vi "核查数据发送(子VI).vi"(8 "错误输入":errorcluster) -> (0 "错误输出":errorcluster)   [LabVIEW 2016, in "数据传输系统.lvlib"]
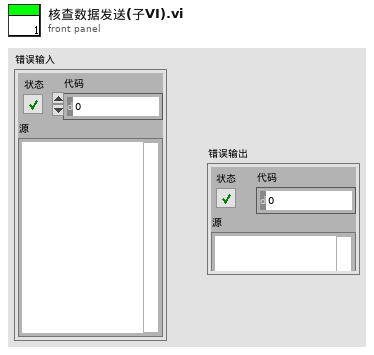
[diagram p1: front panel]
types:
  T1 = enum16{"质控数据", "操作日志", "仪器参数", "系统状态", "运行模式", "测量周期", "超标留样", "报警信息", "环境参数"}
  T2 = enum16{"空白测试", "跨度核查", "标样核查", "加标回收", "平行样", "集成干预"}
  T3 = cluster{"氨氮零点核查索引起始时间":string, "总磷零点核查索引起始时间":string, "总氮零点核查索引起始时间":string, "CODMn零点核查索引起始时间":string, "CODCr零点核查索引起始时间":string, "亚硝酸盐零点核查索引起始时间":string, "硫化物零点核查索引起始时间":string, "ORP零点核查索引起始时间":string}
  T4 = cluster{"[0]":string, "[1]":string, "[2]":string, "[3]":string, "[4]":string, "[5]":string, "[6]":string, "[7]":string}
  T5 = cluster{"PH":string[][], "CODCr":string[][], "氨氮":string[][], "CODMn":string[][], "总氮":string[][], "总磷":string[][], "电导率":string[][], "水温":string[][], "DO":string[][], "浊度":string[][], "叶绿素":string[][], "藻密度":string[][], "铜":string[][], "盐度":string[][], "水位":string[][], "流速":string[][], "瞬时流量":string[][], "累积流量":string[][], "亚硝酸盐":string[][], "硫化物":string[][], "ORP":string[][], "铅":string[][], "镉":string[][], "锌":string[][], "镍":string[][], "锰":string[][], "汞":string[][], "气温":string[][], "气压":string[][], "风速":string[][], "风向":string[][]}
  T6 = cluster{"氨氮跨度核查索引起始时间":string, "总磷跨度核查索引起始时间":string, "总氮跨度核查索引起始时间":string, "CODMn跨度核查索引起始时间":string, "CODCr跨度核查索引起始时间":string, "亚硝酸盐跨度核查索引起始时间":string, "硫化物跨度核查索引起始时间":string, "ORP跨度核查索引起始时间":string}
  T7 = cluster{"氨氮标样核查索引起始时间":string, "总磷标样核查索引起始时间":string, "总氮标样核查索引起始时间":string, "CODMn标样核查索引起始时间":string, "CODCr标样核查索引起始时间":string, "DO标样核查索引起始时间":string, "PH标样核查索引起始时间":string, "比电导率标样核查索引起始时间":string, "水温标样核查索引起始时间":string, "浊度标样核查索引起始时间":string, "叶绿素a标样核查索引起始时间":string, "藻密度标样核查索引起始时间":string, "亚硝酸盐标样核查索引起始时间":string, "硫化物标样核查索引起始时间":string, "ORP标样核查索引起始时间":string}
  T8 = cluster{"[0]":string, "[1]":string, "[2]":string, "[3]":string, "[4]":string, "[5]":string, "[6]":string, "[7]":string, "[8]":string, "[9]":string, "[10]":string, "[11]":string, "[12]":string, "[13]":string, "[14]":string}
  T9 = cluster{"氨氮加标回收索引起始时间":string, "总磷加标回收索引起始时间":string, "总氮加标回收索引起始时间":string, "CODMn加标回收索引起始时间":string, "CODCr加标回收索引起始时间":string}
  T10 = cluster{"[0]":string, "[1]":string, "[2]":string, "[3]":string, "[4]":string}
  T11 = cluster{"氨氮平行样索引起始时间":string, "总磷平行样索引起始时间":string, "总氮平行样索引起始时间":string, "CODMn平行样索引起始时间":string, "CODCr平行样索引起始时间":string}
  T12 = cluster{"氨氮集成干预索引起始时间":string, "总磷集成干预索引起始时间":string, "总氮集成干预索引起始时间":string, "CODMn集成干预索引起始时间":string, "CODCr集成干预索引起始时间":string, "DO集成干预索引起始时间":string, "PH集成干预索引起始时间":string, "比电导率集成干预索引起始时间":string, "水温集成干预索引起始时间":string, "浊度集成干预索引起始时间":string, "叶绿素a集成干预索引起始时间":string, "藻密度集成干预索引起始时间":string, "亚硝酸盐集成干预索引起始时间":string, "硫化物集成干预索引起始时间":string, "ORP集成干预索引起始时间":string}
  T13 = cluster{"氨氮仪器日志索引起始时间":string, "总磷仪器日志索引起始时间":string, "总氮仪器日志索引起始时间":string, "CODMn仪器日志索引起始时间":string, "CODCr仪器日志索引起始时间":string, "系统仪器日志索引起始时间":string}
  T14 = cluster{"[0]":string, "[1]":string, "[2]":string, "[3]":string, "[4]":string, "[5]":string}
  T15 = cluster{"氨氮仪器参数索引起始时间":string, "总磷仪器参数索引起始时间":string, "总氮仪器参数索引起始时间":string, "CODMn仪器参数索引起始时间":string, "CODCr仪器参数索引起始时间":string, "DO仪器参数索引起始时间":string, "PH仪器参数索引起始时间":string, "比电导率仪器参数索引起始时间":string, "水温仪器参数索引起始时间":string, "浊度仪器参数索引起始时间":string, "叶绿素a仪器参数索引起始时间":string, "藻密度仪器参数索引起始时间":string, "ORP仪器参数索引起始时间":string}
  T16 = cluster{"[0]":string, "[1]":string, "[2]":string, "[3]":string, "[4]":string, "[5]":string, "[6]":string, "[7]":string, "[8]":string, "[9]":string, "[10]":string, "[11]":string, "[12]":string}
  T17 = cluster{"氨氮报警信息索引起始时间":string, "总磷报警信息索引起始时间":string, "总氮报警信息索引起始时间":string, "CODMn报警信息索引起始时间":string, "CODCr报警信息索引起始时间":string, "DO报警信息索引起始时间":string, "PH报警信息索引起始时间":string, "比电导率报警信息索引起始时间":string, "水温报警信息索引起始时间":string, "浊度报警信息索引起始时间":string, "叶绿素报警信息索引起始时间":string, "系统报警信息索引起始时间":string}
  T18 = cluster{"[0]":string, "[1]":string, "[2]":string, "[3]":string, "[4]":string, "[5]":string, "[6]":string, "[7]":string, "[8]":string, "[9]":string, "[10]":string, "[11]":string}
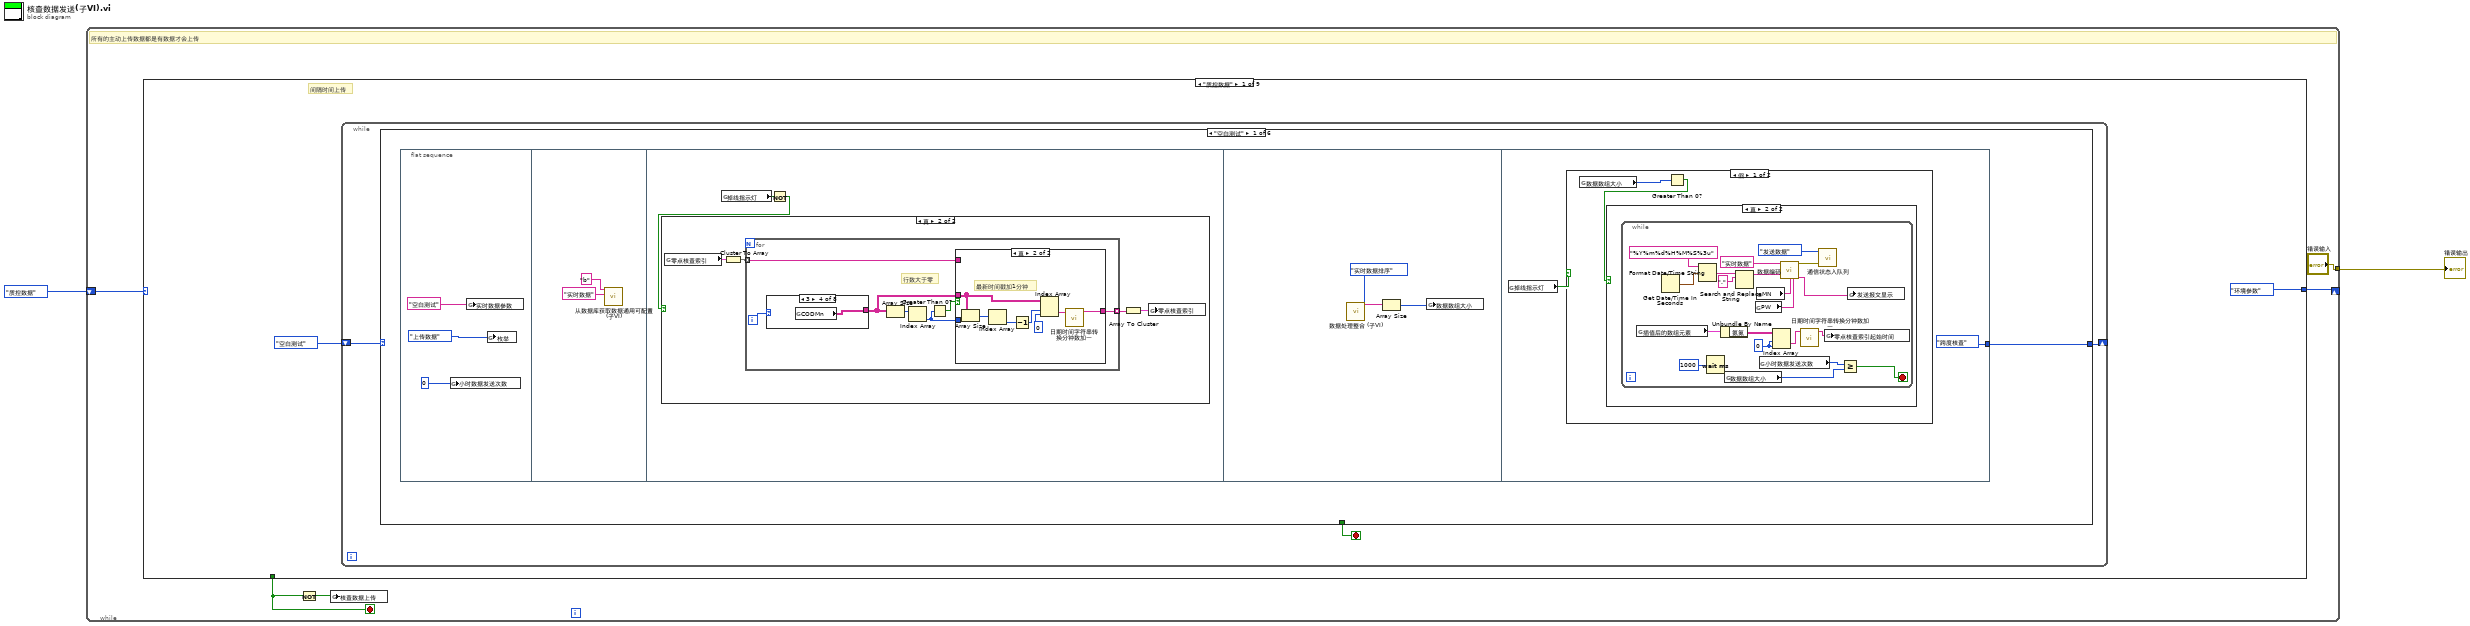
[diagram p0: block diagram]
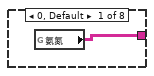
[diagram p3: hidden frame]
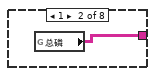
[diagram p4: hidden frame]
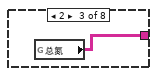
[diagram p5: hidden frame]
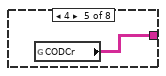
[diagram p6: hidden frame]
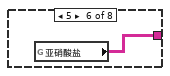
[diagram p7: hidden frame]
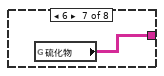
[diagram p8: hidden frame]
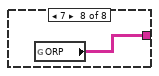
[diagram p9: hidden frame]
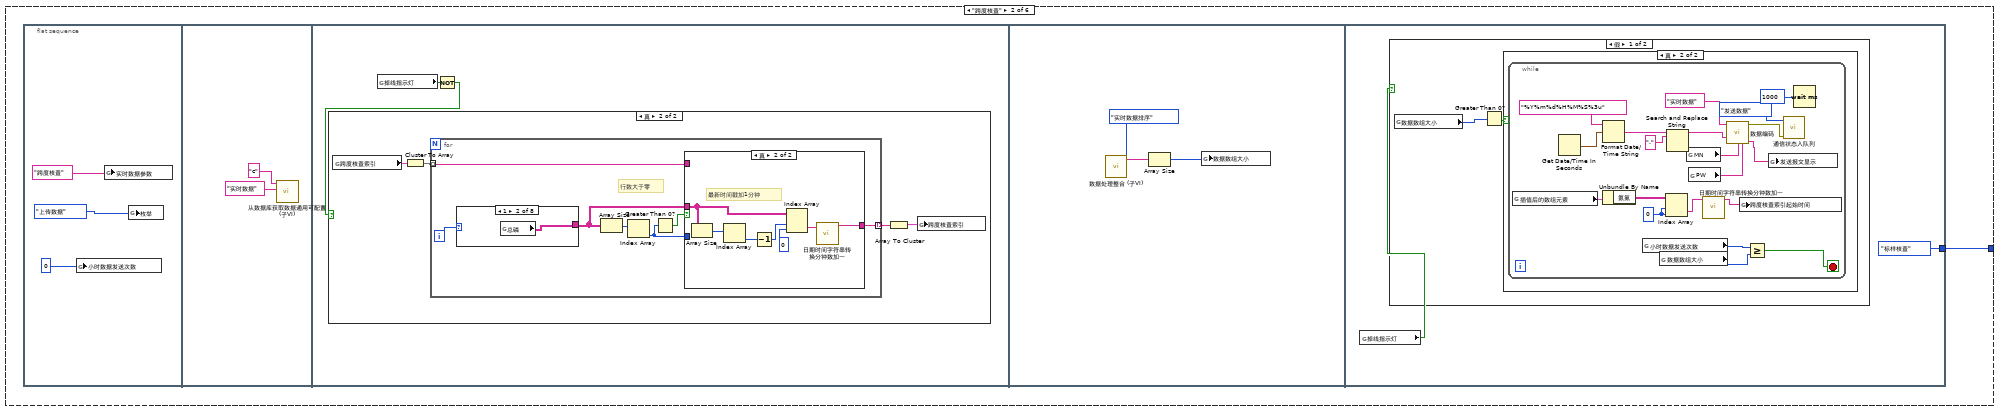
[diagram p13: hidden frame]
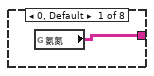
[diagram p15: hidden frame]
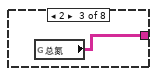
[diagram p16: hidden frame]
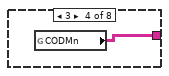
[diagram p17: hidden frame]
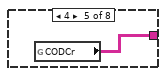
[diagram p18: hidden frame]
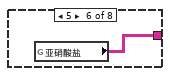
[diagram p19: hidden frame]
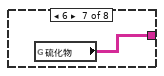
[diagram p20: hidden frame]
diagram:
  n1 = while "While循环" {
    shift-right: [w6] -> _
    shift-left: T1."质控数据" -> [w7]
    tunnel: ["错误输入"] -> w1
    stop <- w4 stop-if-true
    # "所有的主动上传数据都是有数据才会上传"
    n2 = case shown="\"质控数据\"" w7 {
      tunnel: [T1."环境参数" T1."仪器参数" T1."系统状态" T1."运行模式" T1."测量周期" T1."超标留样" T1."报警信息" T1."环境参数" T1."环境参数"] -> w6
      tunnel: [_ _ _ _ _ _ _ _ TRUE] -> w4
      frame "质控数据" {
        # "间隔时间上传"
        n3 = while {
          shift-right: [w10] -> _
          shift-left: T2."空白测试" -> [w11]
          stop <- w12 stop-if-true
          n4 = case shown="\"空白测试\"" w11 {
            tunnel: [_ _ _ _ _ TRUE] -> w12
            tunnel: [w13 w75 w137 w206 w267 w321] -> w10
            frame "空白测试" {
              n5 = flat-sequence {
                tunnel: [T2."跨度核查"] -> w13
                frame #0 {
                  n6 = global write "全局 小时数据发送次数.vi" "小时数据发送次数"(0 ("小时数据发送次数")) -> ()
                  n7 = global write "全局 实时数据参数.vi" "实时数据参数"("空白测试") -> ()
                  n8 = global write "全局1.vi" "枚举"(enum16{"返回请求应答", "上传数据", "返回执行结果"}."上传数据" ("枚举")) -> ()
                }
                frame #1 {
                  n9 = call "从数据库获取数据通用可配置(子VI).vi"("table输入"="实时数据" ("新元素/子数组"), "列队名（唯一）"="b") -> ()  [unwired: 8 in, 2 out]
                }
                frame #2 {
                  n10 = global read "全局 数据发送重叠.vi" "掉线指示灯"() -> (w20:bool)
                  n11 = Not(x=w20) -> (.not. x?=w19:bool)
                  n12 = case shown="真" w19 {
                    frame False {
                    }
                    frame True {
                      n13 = global read "全局 时间2.vi" "零点核查索引"() -> (w24:T3)
                      n14 = Cluster To Array(cluster=w24) -> (array=w23:string[])
                      n15 = for {
                        tunnel: [w26] -> w22 mode=indexing
                        tunnel: w23 -> [w25] mode=indexing
                        i -> [w27]
                        # "行数大于零"
                        n16 = case shown="3" w27 {
                          tunnel: [w32 w33 w34 w35 w36 w37 w38 w39] -> w28
                          frame 0, Default {
                            n17 = global read "全局 所有参数.vi" "氨氮"() -> (w32:string[][])
                          }
                          frame 1 {
                            n18 = global read "全局 所有参数.vi" "总磷"() -> (w33:string[][])
                          }
                          frame 2 {
                            n19 = global read "全局 所有参数.vi" "总氮"() -> (w34:string[][])
                          }
                          frame 3 {
                            n20 = global read "全局 所有参数.vi" "CODMn"() -> (w35:string[][])
                          }
                          frame 4 {
                            n21 = global read "全局 所有参数.vi" "CODCr"() -> (w36:string[][])
                          }
                          frame 5 {
                            n22 = global read "全局 所有参数.vi" "亚硝酸盐"() -> (w37:string[][])
                          }
                          frame 6 {
                            n23 = global read "全局 所有参数.vi" "硫化物"() -> (w38:string[][])
                          }
                          frame 7 {
                            n24 = global read "全局 所有参数.vi" "ORP"() -> (w39:string[][])
                          }
                        }
                        n25 = Array Size(array=w28) -> (size(s)=w30:i32[])
                        n26 = Index Array(array=w30) -> (element=w29:i32)  [unwired: 1 in]
                        n27 = Greater Than 0?(x=w29) -> (x > 0?=w31:bool)
                        n28 = case shown="真" w31 {
                          tunnel: w29 -> [_ _]
                          tunnel: w28 -> [_ w43]
                          tunnel: [w40 w41] -> w26
                          tunnel: w25 -> [w40 _]
                          frame False {
                          }
                          frame True {
                            # "最新时间戳加1分钟"
                            n29 = Array Size(array=w43) -> (size(s)=w46:i32[])
                            n30 = Index Array(array=w46) -> (element=w45:i32)  [unwired: 1 in]
                            n31 = Decrement(x=w45) -> (x-1=w44:i32)
                            n32 = Index Array(array=w43, index (row)=w44, index (col)=0 ("禁用的索引 (列)")) -> (element=w47:string)
                            n33 = call "日期时间字符串转换分钟数加一.vi"("data[0]"=w47) -> ("日期/时间字符串"=w41:string)  [unwired: 10 in]
                          }
                        }
                      }
                      n34 = Array To Cluster(array=w22) -> (cluster=w21:T4)
                      n35 = global write "全局 时间2.vi" "零点核查索引"(w21) -> ()
                    }
                  }
                }
                frame #3 {
                  n36 = call "数据处理整合 (子VI).vi"("枚举"=enum16{"实时数据排序", "小时数据排序"}."实时数据排序") -> ("已排序的数组"=w50:string[])  [unwired: 10 in]
                  n37 = Array Size(array=w50) -> (size(s)=w49:i32)
                  n38 = global write "全局 数据数组大小.vi" "数据数组大小"(w49) -> ()
                }
                frame #4 {
                  n39 = global read "全局 数据发送重叠.vi" "掉线指示灯"() -> (w52:bool)
                  n40 = case shown="假" w52 {
                    frame False {
                      n41 = global read "全局 数据数组大小.vi" "数据数组大小"() -> (w54:i32)
                      n42 = Greater Than 0?(x=w54) -> (x > 0?=w53:bool)
                      n43 = case shown="真" w53 {
                        frame False {
                        }
                        frame True {
                          n44 = while {
                            stop <- w60 stop-if-true
                            w69 = 0 ("禁用的索引 (列)")
                            n45 = global read "插值后的新数组.vi" "插值后的数组元素"() -> (w73:T5)
                            n46 = Get Date/Time In Seconds() -> (seconds since 1Jan1904=w58:timestamp)
                            n47 = Format Date/Time String(time format string (%c)="%Y%m%d%H%M%S%3u" ("时间格式字符串(%c)"), seconds (now)=w58) -> (date/time string=w57:string)  [unwired: 1 in]
                            n48 = Wait (ms)(milliseconds to wait=u32 1000 ("等待时间（毫秒）")) -> ()  [unwired: 1 out]
                            n49 = Unbundle By Name(w73) -> ("氨氮"=w72:string[][])
                            n50 = global read "全局 数据数组大小.vi" "数据数组大小"() -> (w63:i32)
                            n51 = Search and Replace String(input string=w57, search string="." ("搜索字符串")) -> (result string=w55:string)  [unwired: 6 in, 3 out]
                            n52 = global read "断电保存全局.vi" "PW"() -> (w65:string)
                            n53 = global read "断电保存全局.vi" "MN"() -> (w66:string)
                            n54 = global read "全局 小时数据发送次数.vi" "小时数据发送次数"() -> (w61:i32)
                            n55 = Index Array(array=w72, index (row)=w69, index (col)=w69) -> (element=w71:string)
                            n56 = call "数据编码.vi"("table输入"="实时数据" ("新元素/子数组"), "QN"=w55, "MN"=w66, "PW"=w65) -> ("错误常量"=w64:errorcluster, "通讯包字符串"=w68:string)  [unwired: 10 in]
                            n57 = call "日期时间字符串转换分钟数加一.vi"("data[0]"=w71) -> ("日期/时间字符串"=w70:string)  [unwired: 10 in]
                            n58 = call "通信状态入队列.vi"("错误输入（无错误）"=w64, "枚举"=enum16{"打开连接", "发送数据", "读取数据", "数据处理", "关闭连接"}."发送数据") -> ()  [unwired: 9 in, 1 out]
                            n59 = global write "全局 时间2.vi" "零点核查索引起始时间"(w70) -> ()
                            n60 = Greater Or Equal?(x=w61, y=w63) -> (x >= y?=w60:bool)
                            n61 = global write "全局1.vi" "发送报文显示"(w68) -> ()
                          }
                        }
                      }
                    }
                    frame True {
                    }
                  }
                }
              }
            }
            frame "跨度核查" {
              n62 = flat-sequence {
                tunnel: [T2."标样核查"] -> w75
                frame #0 {
                  n63 = global write "全局 小时数据发送次数.vi" "小时数据发送次数"(0 ("小时数据发送次数")) -> ()
                  n64 = global write "全局 实时数据参数.vi" "实时数据参数"("跨度核查") -> ()
                  n65 = global write "全局1.vi" "枚举"(enum16{"返回请求应答", "上传数据", "返回执行结果"}."上传数据" ("枚举")) -> ()
                }
                frame #1 {
                  n66 = call "从数据库获取数据通用可配置(子VI).vi"("table输入"="实时数据" ("新元素/子数组"), "列队名（唯一）"="c") -> ()  [unwired: 8 in, 2 out]
                }
                frame #2 {
                  n67 = global read "全局 数据发送重叠.vi" "掉线指示灯"() -> (w82:bool)
                  n68 = Not(x=w82) -> (.not. x?=w81:bool)
                  n69 = case shown="真" w81 {
                    frame False {
                    }
                    frame True {
                      n70 = global read "全局 时间2.vi" "跨度核查索引"() -> (w86:T6)
                      n71 = Cluster To Array(cluster=w86) -> (array=w85:string[])
                      n72 = for {
                        tunnel: [w88] -> w84 mode=indexing
                        tunnel: w85 -> [w87] mode=indexing
                        i -> [w89]
                        # "行数大于零"
                        n73 = case shown="1" w89 {
                          tunnel: [w94 w95 w96 w97 w98 w99 w100 w101] -> w90
                          frame 0, Default {
                            n74 = global read "全局 所有参数.vi" "氨氮"() -> (w94:string[][])
                          }
                          frame 1 {
                            n75 = global read "全局 所有参数.vi" "总磷"() -> (w95:string[][])
                          }
                          frame 2 {
                            n76 = global read "全局 所有参数.vi" "总氮"() -> (w96:string[][])
                          }
                          frame 3 {
                            n77 = global read "全局 所有参数.vi" "CODMn"() -> (w97:string[][])
                          }
                          frame 4 {
                            n78 = global read "全局 所有参数.vi" "CODCr"() -> (w98:string[][])
                          }
                          frame 5 {
                            n79 = global read "全局 所有参数.vi" "亚硝酸盐"() -> (w99:string[][])
                          }
                          frame 6 {
                            n80 = global read "全局 所有参数.vi" "硫化物"() -> (w100:string[][])
                          }
                          frame 7 {
                            n81 = global read "全局 所有参数.vi" "ORP"() -> (w101:string[][])
                          }
                        }
                        n82 = Array Size(array=w90) -> (size(s)=w92:i32[])
                        n83 = Index Array(array=w92) -> (element=w91:i32)  [unwired: 1 in]
                        n84 = Greater Than 0?(x=w91) -> (x > 0?=w93:bool)
                        n85 = case shown="真" w93 {
                          tunnel: w91 -> [_ _]
                          tunnel: w90 -> [_ w105]
                          tunnel: [w102 w103] -> w88
                          tunnel: w87 -> [w102 _]
                          frame False {
                          }
                          frame True {
                            # "最新时间戳加1分钟"
                            n86 = Array Size(array=w105) -> (size(s)=w108:i32[])
                            n87 = Index Array(array=w108) -> (element=w107:i32)  [unwired: 1 in]
                            n88 = Decrement(x=w107) -> (x-1=w106:i32)
                            n89 = Index Array(array=w105, index (row)=w106, index (col)=0 ("禁用的索引 (列)")) -> (element=w109:string)
                            n90 = call "日期时间字符串转换分钟数加一.vi"("data[0]"=w109) -> ("日期/时间字符串"=w103:string)  [unwired: 10 in]
                          }
                        }
                      }
                      n91 = Array To Cluster(array=w84) -> (cluster=w83:T4)
                      n92 = global write "全局 时间2.vi" "跨度核查索引"(w83) -> ()
                    }
                  }
                }
                frame #3 {
                  n93 = call "数据处理整合 (子VI).vi"("枚举"=enum16{"实时数据排序", "小时数据排序"}."实时数据排序") -> ("已排序的数组"=w112:string[])  [unwired: 10 in]
                  n94 = Array Size(array=w112) -> (size(s)=w111:i32)
                  n95 = global write "全局 数据数组大小.vi" "数据数组大小"(w111) -> ()
                }
                frame #4 {
                  n96 = global read "全局 数据发送重叠.vi" "掉线指示灯"() -> (w114:bool)
                  n97 = case shown="假" w114 {
                    frame False {
                      n98 = global read "全局 数据数组大小.vi" "数据数组大小"() -> (w116:i32)
                      n99 = Greater Than 0?(x=w116) -> (x > 0?=w115:bool)
                      n100 = case shown="真" w115 {
                        frame False {
                        }
                        frame True {
                          n101 = while {
                            stop <- w122 stop-if-true
                            w131 = 0 ("禁用的索引 (列)")
                            n102 = global read "插值后的新数组.vi" "插值后的数组元素"() -> (w135:T5)
                            n103 = Get Date/Time In Seconds() -> (seconds since 1Jan1904=w120:timestamp)
                            n104 = Format Date/Time String(time format string (%c)="%Y%m%d%H%M%S%3u" ("时间格式字符串(%c)"), seconds (now)=w120) -> (date/time string=w119:string)  [unwired: 1 in]
                            n105 = Unbundle By Name(w135) -> ("氨氮"=w134:string[][])
                            n106 = global read "全局 小时数据发送次数.vi" "小时数据发送次数"() -> (w123:i32)
                            n107 = global read "全局 数据数组大小.vi" "数据数组大小"() -> (w124:i32)
                            n108 = Index Array(array=w134, index (row)=w131, index (col)=w131) -> (element=w133:string)
                            n109 = Search and Replace String(input string=w119, search string="." ("搜索字符串")) -> (result string=w117:string)  [unwired: 6 in, 3 out]
                            n110 = global read "断电保存全局.vi" "MN"() -> (w129:string)
                            n111 = global read "断电保存全局.vi" "PW"() -> (w128:string)
                            n112 = call "日期时间字符串转换分钟数加一.vi"("data[0]"=w133) -> ("日期/时间字符串"=w132:string)  [unwired: 10 in]
                            n113 = call "数据编码.vi"("table输入"="实时数据" ("新元素/子数组"), "QN"=w117, "MN"=w129, "PW"=w128) -> ("错误常量"=w126:errorcluster, "通讯包字符串"=w127:string)  [unwired: 10 in]
                            n114 = global write "全局 时间2.vi" "跨度核查索引起始时间"(w132) -> ()
                            n115 = Greater Or Equal?(x=w123, y=w124) -> (x >= y?=w122:bool)
                            n116 = global write "全局1.vi" "发送报文显示"(w127) -> ()
                            n117 = call "通信状态入队列.vi"("错误输入（无错误）"=w126, "枚举"=enum16{"打开连接", "发送数据", "读取数据", "数据处理", "关闭连接"}."发送数据") -> ()  [unwired: 9 in, 1 out]
                            n118 = Wait (ms)(milliseconds to wait=u32 1000 ("等待时间（毫秒）")) -> ()  [unwired: 1 out]
                          }
                        }
                      }
                    }
                    frame True {
                    }
                  }
                }
              }
            }
            frame "标样核查" {
              n119 = flat-sequence {
                tunnel: [T2."加标回收"] -> w137
                frame #0 {
                  n120 = global write "全局 小时数据发送次数.vi" "小时数据发送次数"(0 ("小时数据发送次数")) -> ()
                  n121 = global write "全局 实时数据参数.vi" "实时数据参数"("核查数据") -> ()
                  n122 = global write "全局1.vi" "枚举"(enum16{"返回请求应答", "上传数据", "返回执行结果"}."上传数据" ("枚举")) -> ()
                }
                frame #1 {
                  n123 = call "从数据库获取数据通用可配置(子VI).vi"("table输入"="实时数据" ("新元素/子数组"), "列队名（唯一）"="n") -> ()  [unwired: 8 in, 2 out]
                }
                frame #2 {
                  n124 = global read "全局 数据发送重叠.vi" "掉线指示灯"() -> (w144:bool)
                  n125 = Not(x=w144) -> (.not. x?=w143:bool)
                  n126 = case shown="真" w143 {
                    frame False {
                    }
                    frame True {
                      n127 = global read "全局 时间2.vi" "标样核查索引"() -> (w148:T7)
                      n128 = Cluster To Array(cluster=w148) -> (array=w147:string[])
                      n129 = for {
                        tunnel: [w150] -> w145 mode=indexing
                        tunnel: w147 -> [w149] mode=indexing
                        i -> [w151]
                        # "行数大于零"
                        n130 = case shown="0, 默认" w151 {
                          tunnel: [w156 w157 w158 w159 w160 w161 w162 w163 w164 w165 w166 w167 w168 w169 w170] -> w152
                          frame 0, Default {
                            n131 = global read "全局 所有参数.vi" "氨氮"() -> (w156:string[][])
                          }
                          frame 1 {
                            n132 = global read "全局 所有参数.vi" "总磷"() -> (w157:string[][])
                          }
                          frame 2 {
                            n133 = global read "全局 所有参数.vi" "总氮"() -> (w158:string[][])
                          }
                          frame 3 {
                            n134 = global read "全局 所有参数.vi" "CODMn"() -> (w159:string[][])
                          }
                          frame 4 {
                            n135 = global read "全局 所有参数.vi" "CODCr"() -> (w160:string[][])
                          }
                          frame 5 {
                            n136 = global read "全局 所有参数.vi" "DO"() -> (w161:string[][])
                          }
                          frame 6 {
                            n137 = global read "全局 所有参数.vi" "PH"() -> (w162:string[][])
                          }
                          frame 7 {
                            n138 = global read "全局 所有参数.vi" "电导率"() -> (w163:string[][])
                          }
                          frame 8 {
                            n139 = global read "全局 所有参数.vi" "水温"() -> (w164:string[][])
                          }
                          frame 9 {
                            n140 = global read "全局 所有参数.vi" "浊度"() -> (w165:string[][])
                          }
                          frame 10 {
                            n141 = global read "全局 所有参数.vi" "叶绿素"() -> (w166:string[][])
                          }
                          frame 11 {
                            n142 = global read "全局 所有参数.vi" "藻密度"() -> (w167:string[][])
                          }
                          frame 12 {
                            n143 = global read "全局 所有参数.vi" "亚硝酸盐"() -> (w168:string[][])
                          }
                          frame 13 {
                            n144 = global read "全局 所有参数.vi" "硫化物"() -> (w169:string[][])
                          }
                          frame 14 {
                            n145 = global read "全局 所有参数.vi" "ORP"() -> (w170:string[][])
                          }
                        }
                        n146 = Array Size(array=w152) -> (size(s)=w154:i32[])
                        n147 = Index Array(array=w154) -> (element=w153:i32)  [unwired: 1 in]
                        n148 = Greater Than 0?(x=w153) -> (x > 0?=w155:bool)
                        n149 = case shown="真" w155 {
                          tunnel: w151 -> [_ _]
                          tunnel: w153 -> [_ _]
                          tunnel: w152 -> [_ w173]
                          tunnel: [w171 w172] -> w150
                          tunnel: w149 -> [w171 _]
                          frame False {
                          }
                          frame True {
                            # "最新时间戳加1分钟"
                            n150 = Array Size(array=w173) -> (size(s)=w177:i32[])
                            n151 = Index Array(array=w177) -> (element=w176:i32)  [unwired: 1 in]
                            n152 = Decrement(x=w176) -> (x-1=w175:i32)
                            n153 = Index Array(array=w173, index (row)=w175, index (col)=0 ("禁用的索引 (列)")) -> (element=w178:string)
                            n154 = call "日期时间字符串转换分钟数加一.vi"("data[0]"=w178) -> ("日期/时间字符串"=w172:string)  [unwired: 10 in]
                          }
                        }
                      }
                      n155 = Array To Cluster(array=w145) -> (cluster=w146:T8)
                      n156 = global write "全局 时间2.vi" "标样核查索引"(w146) -> ()
                    }
                  }
                }
                frame #3 {
                  n157 = call "数据处理整合 (子VI).vi"("枚举"=enum16{"实时数据排序", "小时数据排序"}."实时数据排序") -> ("已排序的数组"=w181:string[])  [unwired: 10 in]
                  n158 = Array Size(array=w181) -> (size(s)=w180:i32)
                  n159 = global write "全局 数据数组大小.vi" "数据数组大小"(w180) -> ()
                }
                frame #4 {
                  n160 = global read "全局 数据发送重叠.vi" "掉线指示灯"() -> (w183:bool)
                  n161 = case shown="假" w183 {
                    frame False {
                      n162 = global read "全局 数据数组大小.vi" "数据数组大小"() -> (w185:i32)
                      n163 = Greater Than 0?(x=w185) -> (x > 0?=w184:bool)
                      n164 = case shown="真" w184 {
                        frame False {
                        }
                        frame True {
                          n165 = while {
                            stop <- w192 stop-if-true
                            w200 = 0 ("禁用的索引 (列)")
                            n166 = global read "插值后的新数组.vi" "插值后的数组元素"() -> (w204:T5)
                            n167 = Get Date/Time In Seconds() -> (seconds since 1Jan1904=w189:timestamp)
                            n168 = Format Date/Time String(time format string (%c)="%Y%m%d%H%M%S%3u" ("时间格式字符串(%c)"), seconds (now)=w189) -> (date/time string=w188:string)  [unwired: 1 in]
                            n169 = Unbundle By Name(w204) -> ("氨氮"=w203:string[][])
                            n170 = global read "全局 小时数据发送次数.vi" "小时数据发送次数"() -> (w193:i32)
                            n171 = global read "断电保存全局.vi" "MN"() -> (w197:string)
                            n172 = Search and Replace String(input string=w188, search string="." ("搜索字符串")) -> (result string=w186:string)  [unwired: 6 in, 3 out]
                            n173 = global read "断电保存全局.vi" "PW"() -> (w196:string)
                            n174 = global read "全局 数据数组大小.vi" "数据数组大小"() -> (w194:i32)
                            n175 = Index Array(array=w203, index (row)=w200, index (col)=w200) -> (element=w202:string)
                            n176 = call "日期时间字符串转换分钟数加一.vi"("data[0]"=w202) -> ("日期/时间字符串"=w201:string)  [unwired: 10 in]
                            n177 = call "数据编码.vi"("table输入"="实时数据" ("新元素/子数组"), "QN"=w186, "MN"=w197, "PW"=w196) -> ("错误常量"=w195:errorcluster, "通讯包字符串"=w199:string)  [unwired: 10 in]
                            n178 = global write "全局 时间2.vi" "标样核查索引起始时间"(w201) -> ()
                            n179 = global write "全局1.vi" "发送报文显示"(w199) -> ()
                            n180 = Greater Or Equal?(x=w193, y=w194) -> (x >= y?=w192:bool)
                            n181 = call "通信状态入队列.vi"("错误输入（无错误）"=w195, "枚举"=enum16{"打开连接", "发送数据", "读取数据", "数据处理", "关闭连接"}."发送数据") -> ()  [unwired: 9 in, 1 out]
                            n182 = Wait (ms)(milliseconds to wait=u32 1000 ("等待时间（毫秒）")) -> ()  [unwired: 1 out]
                          }
                        }
                      }
                    }
                    frame True {
                    }
                  }
                }
              }
            }
            frame "加标回收" {
              n183 = flat-sequence {
                tunnel: [T2."平行样"] -> w206
                frame #0 {
                  n184 = global write "全局 小时数据发送次数.vi" "小时数据发送次数"(0 ("小时数据发送次数")) -> ()
                  n185 = global write "全局 实时数据参数.vi" "实时数据参数"("加标回收测试") -> ()
                  n186 = global write "全局1.vi" "枚举"(enum16{"返回请求应答", "上传数据", "返回执行结果"}."上传数据" ("枚举")) -> ()
                }
                frame #1 {
                  n187 = call "从数据库获取数据通用可配置(子VI).vi"("table输入"="加标回收" ("新元素/子数组"), "列队名（唯一）"="d") -> ()  [unwired: 8 in, 2 out]
                }
                frame #2 {
                  n188 = global read "全局 数据发送重叠.vi" "掉线指示灯"() -> (w213:bool)
                  n189 = Not(x=w213) -> (.not. x?=w212:bool)
                  n190 = case shown="真" w212 {
                    frame False {
                    }
                    frame True {
                      n191 = global read "全局 时间2.vi" "加标回收索引"() -> (w217:T9)
                      n192 = Cluster To Array(cluster=w217) -> (array=w216:string[])
                      n193 = for {
                        tunnel: [w219] -> w214 mode=indexing
                        tunnel: w216 -> [w218] mode=indexing
                        i -> [w220]
                        # "行数大于零"
                        n194 = case shown="0, 默认" w220 {
                          tunnel: [w225 w226 w227 w228 w229] -> w221
                          frame 0, Default {
                            n195 = global read "全局 所有参数.vi" "氨氮加标回收率"() -> (w225:string[][])
                          }
                          frame 1 {
                            n196 = global read "全局 所有参数.vi" "总磷加标回收率"() -> (w226:string[][])
                          }
                          frame 2 {
                            n197 = global read "全局 所有参数.vi" "总氮加标回收率"() -> (w227:string[][])
                          }
                          frame 3 {
                            n198 = global read "全局 所有参数.vi" "CODMn加标回收率"() -> (w228:string[][])
                          }
                          frame 4 {
                            n199 = global read "全局 所有参数.vi" "CODCr加标回收率"() -> (w229:string[][])
                          }
                        }
                        n200 = Array Size(array=w221) -> (size(s)=w223:i32[])
                        n201 = Index Array(array=w223) -> (element=w222:i32)  [unwired: 1 in]
                        n202 = Greater Than 0?(x=w222) -> (x > 0?=w224:bool)
                        n203 = case shown="真" w224 {
                          tunnel: w220 -> [_ _]
                          tunnel: w222 -> [_ _]
                          tunnel: w221 -> [_ w234]
                          tunnel: [w230 w231] -> w219
                          tunnel: w218 -> [w230 _]
                          frame False {
                          }
                          frame True {
                            # "最新时间戳加1分钟"
                            n204 = Array Size(array=w234) -> (size(s)=w236:i32[])
                            n205 = Index Array(array=w236) -> (element=w235:i32)  [unwired: 1 in]
                            n206 = Decrement(x=w235) -> (x-1=w233:i32)
                            n207 = Index Array(array=w234, index (row)=w233, index (col)=0 ("禁用的索引 (列)")) -> (element=w237:string)
                            n208 = call "日期时间字符串转换分钟数加一.vi"("data[0]"=w237) -> ("日期/时间字符串"=w231:string)  [unwired: 10 in]
                          }
                        }
                      }
                      n209 = Array To Cluster(array=w214) -> (cluster=w215:T10)
                      n210 = global write "全局 时间2.vi" "加标回收索引"(w215) -> ()
                    }
                  }
                }
                frame #3 {
                  n211 = call "加标回收数据处理整合 (子VI).vi"("枚举"=enum16{"实时数据排序", "小时数据排序"}."实时数据排序") -> ("已排序的数组"=w239:string[])  [unwired: 10 in]
                  n212 = Array Size(array=w239) -> (size(s)=w240:i32)
                  n213 = global write "全局 数据数组大小.vi" "数据数组大小"(w240) -> ()
                }
                frame #4 {
                  n214 = global read "全局 数据发送重叠.vi" "掉线指示灯"() -> (w242:bool)
                  n215 = case shown="假" w242 {
                    frame False {
                      n216 = global read "全局 数据数组大小.vi" "数据数组大小"() -> (w244:i32)
                      n217 = Greater Than 0?(x=w244) -> (x > 0?=w243:bool)
                      n218 = case shown="真" w243 {
                        frame False {
                        }
                        frame True {
                          n219 = while {
                            stop <- w251 stop-if-true
                            n220 = global read "全局 数据数组大小.vi" "数据数组大小"() -> (w262:i32)
                            n221 = global read "插值后的新数组.vi" "插值后的数组元素"() -> (w265:T5)
                            n222 = Get Date/Time In Seconds() -> (seconds since 1Jan1904=w248:timestamp)
                            n223 = Format Date/Time String(time format string (%c)="%Y%m%d%H%M%S%3u" ("时间格式字符串(%c)"), seconds (now)=w248) -> (date/time string=w247:string)  [unwired: 1 in]
                            n224 = Decrement(x=w262) -> (x-1=w261:i32)
                            n225 = Unbundle By Name(w265) -> ("氨氮"=w264:string[][])
                            n226 = Search and Replace String(input string=w247, search string="." ("搜索字符串")) -> (result string=w245:string)  [unwired: 6 in, 3 out]
                            n227 = global read "全局 小时数据发送次数.vi" "小时数据发送次数"() -> (w252:i32)
                            n228 = global read "断电保存全局.vi" "MN"() -> (w256:string)
                            n229 = Index Array(array=w264, index (row)=w261, index (col)=0 ("禁用的索引 (列)")) -> (element=w260:string)
                            n230 = global read "断电保存全局.vi" "PW"() -> (w255:string)
                            n231 = global read "全局 数据数组大小.vi" "数据数组大小"() -> (w253:i32)
                            n232 = call "日期时间字符串转换分钟数加一.vi"("data[0]"=w260) -> ("日期/时间字符串"=w259:string)  [unwired: 10 in]
                            n233 = call "数据编码.vi"("table输入"="实时数据" ("新元素/子数组"), "QN"=w245, "MN"=w256, "PW"=w255) -> ("错误常量"=w254:errorcluster, "通讯包字符串"=w258:string)  [unwired: 10 in]
                            n234 = global write "全局 时间2.vi" "加标回收索引起始时间"(w259) -> ()
                            n235 = Greater Or Equal?(x=w252, y=w253) -> (x >= y?=w251:bool)
                            n236 = global write "全局1.vi" "发送报文显示"(w258) -> ()
                            n237 = call "通信状态入队列.vi"("错误输入（无错误）"=w254, "枚举"=enum16{"打开连接", "发送数据", "读取数据", "数据处理", "关闭连接"}."发送数据") -> ()  [unwired: 9 in, 1 out]
                            n238 = Wait (ms)(milliseconds to wait=u32 1000 ("等待时间（毫秒）")) -> ()  [unwired: 1 out]
                          }
                        }
                      }
                    }
                    frame True {
                    }
                  }
                }
              }
            }
            frame "平行样" {
              n239 = flat-sequence {
                tunnel: [T2."集成干预"] -> w267
                frame #0 {
                  n240 = global write "全局 小时数据发送次数.vi" "小时数据发送次数"(0 ("小时数据发送次数")) -> ()
                  n241 = global write "全局 实时数据参数.vi" "实时数据参数"("平行样测试") -> ()
                  n242 = global write "全局1.vi" "枚举"(enum16{"返回请求应答", "上传数据", "返回执行结果"}."上传数据" ("枚举")) -> ()
                }
                frame #1 {
                  n243 = call "从数据库获取数据通用可配置(子VI).vi"("table输入"="平行样测试" ("新元素/子数组"), "列队名（唯一）"="e") -> ()  [unwired: 8 in, 2 out]
                }
                frame #2 {
                  n244 = global read "全局 数据发送重叠.vi" "掉线指示灯"() -> (w274:bool)
                  n245 = Not(x=w274) -> (.not. x?=w273:bool)
                  n246 = case shown="真" w273 {
                    frame False {
                    }
                    frame True {
                      n247 = global read "全局 时间2.vi" "平行样索引"() -> (w278:T11)
                      n248 = Cluster To Array(cluster=w278) -> (array=w277:string[])
                      n249 = for {
                        tunnel: [w280] -> w275 mode=indexing
                        tunnel: w277 -> [w279] mode=indexing
                        i -> [w281]
                        # "行数大于零"
                        n250 = case shown="4" w281 {
                          tunnel: [w286 w287 w288 w289 w290] -> w282
                          frame 0, Default {
                            n251 = global read "全局 所有参数.vi" "氨氮"() -> (w286:string[][])
                          }
                          frame 1 {
                            n252 = global read "全局 所有参数.vi" "总磷"() -> (w287:string[][])
                          }
                          frame 2 {
                            n253 = global read "全局 所有参数.vi" "总氮"() -> (w288:string[][])
                          }
                          frame 3 {
                            n254 = global read "全局 所有参数.vi" "CODMn"() -> (w289:string[][])
                          }
                          frame 4 {
                            n255 = global read "全局 所有参数.vi" "CODCr"() -> (w290:string[][])
                          }
                        }
                        n256 = Array Size(array=w282) -> (size(s)=w284:i32[])
                        n257 = Index Array(array=w284) -> (element=w283:i32)  [unwired: 1 in]
                        n258 = Greater Than 0?(x=w283) -> (x > 0?=w285:bool)
                        n259 = case shown="真" w285 {
                          tunnel: w281 -> [_ _]
                          tunnel: w283 -> [_ _]
                          tunnel: w282 -> [_ w295]
                          tunnel: [w291 w292] -> w280
                          tunnel: w279 -> [w291 _]
                          frame False {
                          }
                          frame True {
                            # "最新时间戳加1分钟"
                            n260 = Array Size(array=w295) -> (size(s)=w297:i32[])
                            n261 = Index Array(array=w297) -> (element=w296:i32)  [unwired: 1 in]
                            n262 = Decrement(x=w296) -> (x-1=w294:i32)
                            n263 = Index Array(array=w295, index (row)=w294, index (col)=0 ("禁用的索引 (列)")) -> (element=w298:string)
                            n264 = call "日期时间字符串转换分钟数加一.vi"("data[0]"=w298) -> ("日期/时间字符串"=w292:string)  [unwired: 10 in]
                          }
                        }
                      }
                      n265 = Array To Cluster(array=w275) -> (cluster=w276:T10)
                      n266 = global write "全局 时间2.vi" "平行样索引"(w276) -> ()
                    }
                  }
                }
                frame #3 {
                  n267 = call "数据处理整合 (子VI).vi"("枚举"=enum16{"实时数据排序", "小时数据排序"}."实时数据排序") -> ("已排序的数组"=w301:string[])  [unwired: 10 in]
                  n268 = Array Size(array=w301) -> (size(s)=w300:i32)
                  n269 = global write "全局 数据数组大小.vi" "数据数组大小"(w300) -> ()
                }
                frame #4 {
                  n270 = global read "全局 数据发送重叠.vi" "掉线指示灯"() -> (w302:bool)
                  n271 = case shown="假" w302 {
                    frame False {
                      n272 = global read "全局 数据数组大小.vi" "数据数组大小"() -> (w305:i32)
                      n273 = Greater Than 0?(x=w305) -> (x > 0?=w304:bool)
                      n274 = case shown="真" w304 {
                        frame False {
                        }
                        frame True {
                          n275 = while {
                            stop <- w312 stop-if-true
                            n276 = Get Date/Time In Seconds() -> (seconds since 1Jan1904=w309:timestamp)
                            n277 = Format Date/Time String(time format string (%c)="%Y%m%d%H%M%S%3u" ("时间格式字符串(%c)"), seconds (now)=w309) -> (date/time string=w308:string)  [unwired: 1 in]
                            n278 = global read "全局 小时数据发送次数.vi" "小时数据发送次数"() -> (w313:i32)
                            n279 = global read "全局 数据数组大小.vi" "数据数组大小"() -> (w314:i32)
                            n280 = Search and Replace String(input string=w308, search string="." ("搜索字符串")) -> (result string=w306:string)  [unwired: 6 in, 3 out]
                            n281 = global read "断电保存全局.vi" "MN"() -> (w317:string)
                            n282 = global read "断电保存全局.vi" "PW"() -> (w316:string)
                            n283 = call "数据编码.vi"("table输入"="实时数据" ("新元素/子数组"), "QN"=w306, "MN"=w317, "PW"=w316) -> ("错误常量"=w315:errorcluster, "通讯包字符串"=w319:string)  [unwired: 10 in]
                            n284 = Greater Or Equal?(x=w313, y=w314) -> (x >= y?=w312:bool)
                            n285 = global write "全局1.vi" "发送报文显示"(w319) -> ()
                            n286 = call "通信状态入队列.vi"("错误输入（无错误）"=w315, "枚举"=enum16{"打开连接", "发送数据", "读取数据", "数据处理", "关闭连接"}."发送数据") -> ()  [unwired: 9 in, 1 out]
                            n287 = Wait (ms)(milliseconds to wait=u32 1000 ("等待时间（毫秒）")) -> ()  [unwired: 1 out]
                          }
                        }
                      }
                    }
                    frame True {
                    }
                  }
                }
              }
            }
            frame "集成干预" {
              n288 = flat-sequence {
                tunnel: [T2."集成干预"] -> w321
                frame #0 {
                  n289 = global write "全局 小时数据发送次数.vi" "小时数据发送次数"(0 ("小时数据发送次数")) -> ()
                  n290 = global write "全局 实时数据参数.vi" "实时数据参数"("集成干预测试") -> ()
                  n291 = global write "全局1.vi" "枚举"(enum16{"返回请求应答", "上传数据", "返回执行结果"}."上传数据" ("枚举")) -> ()
                }
                frame #1 {
                  n292 = call "从数据库获取数据通用可配置(子VI).vi"("table输入"="集成干预测试" ("新元素/子数组"), "列队名（唯一）"="f") -> ()  [unwired: 8 in, 2 out]
                }
                frame #2 {
                  n293 = global read "全局 数据发送重叠.vi" "掉线指示灯"() -> (w329:bool)
                  n294 = Not(x=w329) -> (.not. x?=w328:bool)
                  n295 = case shown="真" w328 {
                    frame False {
                    }
                    frame True {
                      n296 = global read "全局 时间2.vi" "集成干预索引"() -> (w333:T12)
                      n297 = Cluster To Array(cluster=w333) -> (array=w332:string[])
                      n298 = for {
                        tunnel: [w335] -> w330 mode=indexing
                        tunnel: w332 -> [w334] mode=indexing
                        i -> [w336]
                        # "行数大于零"
                        n299 = case shown="0, 默认" w336 {
                          tunnel: [w341 w342 w343 w344 w345 w346 w347 w348 w349 w350 w351 w352 w353 w354 w355] -> w337
                          frame 0, Default {
                            n300 = global read "全局 所有参数.vi" "氨氮"() -> (w341:string[][])
                          }
                          frame 1 {
                            n301 = global read "全局 所有参数.vi" "总磷"() -> (w342:string[][])
                          }
                          frame 2 {
                            n302 = global read "全局 所有参数.vi" "总氮"() -> (w343:string[][])
                          }
                          frame 3 {
                            n303 = global read "全局 所有参数.vi" "CODMn"() -> (w344:string[][])
                          }
                          frame 4 {
                            n304 = global read "全局 所有参数.vi" "CODCr"() -> (w345:string[][])
                          }
                          frame 5 {
                            n305 = global read "全局 所有参数.vi" "DO"() -> (w346:string[][])
                          }
                          frame 6 {
                            n306 = global read "全局 所有参数.vi" "PH"() -> (w347:string[][])
                          }
                          frame 7 {
                            n307 = global read "全局 所有参数.vi" "电导率"() -> (w348:string[][])
                          }
                          frame 8 {
                            n308 = global read "全局 所有参数.vi" "水温"() -> (w349:string[][])
                          }
                          frame 9 {
                            n309 = global read "全局 所有参数.vi" "浊度"() -> (w350:string[][])
                          }
                          frame 10 {
                            n310 = global read "全局 所有参数.vi" "叶绿素"() -> (w351:string[][])
                          }
                          frame 11 {
                            n311 = global read "全局 所有参数.vi" "藻密度"() -> (w352:string[][])
                          }
                          frame 12 {
                            n312 = global read "全局 所有参数.vi" "亚硝酸盐"() -> (w353:string[][])
                          }
                          frame 13 {
                            n313 = global read "全局 所有参数.vi" "硫化物"() -> (w354:string[][])
                          }
                          frame 14 {
                            n314 = global read "全局 所有参数.vi" "ORP"() -> (w355:string[][])
                          }
                        }
                        n315 = Array Size(array=w337) -> (size(s)=w339:i32[])
                        n316 = Index Array(array=w339) -> (element=w338:i32)  [unwired: 1 in]
                        n317 = Greater Than 0?(x=w338) -> (x > 0?=w340:bool)
                        n318 = case shown="真" w340 {
                          tunnel: w336 -> [_ _]
                          tunnel: w338 -> [_ _]
                          tunnel: w337 -> [_ w358]
                          tunnel: [w356 w357] -> w335
                          tunnel: w334 -> [w356 _]
                          frame False {
                          }
                          frame True {
                            # "最新时间戳加1分钟"
                            n319 = Array Size(array=w358) -> (size(s)=w362:i32[])
                            n320 = Index Array(array=w362) -> (element=w361:i32)  [unwired: 1 in]
                            n321 = Decrement(x=w361) -> (x-1=w360:i32)
                            n322 = Index Array(array=w358, index (row)=w360, index (col)=0 ("禁用的索引 (列)")) -> (element=w363:string)
                            n323 = call "日期时间字符串转换分钟数加一.vi"("data[0]"=w363) -> ("日期/时间字符串"=w357:string)  [unwired: 10 in]
                          }
                        }
                      }
                      n324 = Array To Cluster(array=w330) -> (cluster=w331:T8)
                      n325 = global write "全局 时间2.vi" "集成干预索引"(w331) -> ()
                    }
                  }
                }
                frame #3 {
                  n326 = call "数据处理整合 (子VI).vi"("枚举"=enum16{"实时数据排序", "小时数据排序"}."实时数据排序") -> ("已排序的数组"=w366:string[])  [unwired: 10 in]
                  n327 = Array Size(array=w366) -> (size(s)=w365:i32)
                  n328 = global write "全局 数据数组大小.vi" "数据数组大小"(w365) -> ()
                }
                frame #4 {
                  n329 = global read "全局 数据发送重叠.vi" "掉线指示灯"() -> (w368:bool)
                  n330 = case shown="假" w368 {
                    frame False {
                      n331 = global read "全局 数据数组大小.vi" "数据数组大小"() -> (w370:i32)
                      n332 = Greater Than 0?(x=w370) -> (x > 0?=w369:bool)
                      n333 = case shown="真" w369 {
                        frame False {
                        }
                        frame True {
                          n334 = while {
                            stop <- w377 stop-if-true
                            n335 = Get Date/Time In Seconds() -> (seconds since 1Jan1904=w374:timestamp)
                            n336 = Format Date/Time String(time format string (%c)="%Y%m%d%H%M%S%3u" ("时间格式字符串(%c)"), seconds (now)=w374) -> (date/time string=w373:string)  [unwired: 1 in]
                            n337 = global read "全局 数据数组大小.vi" "数据数组大小"() -> (w379:i32)
                            n338 = global read "全局 小时数据发送次数.vi" "小时数据发送次数"() -> (w378:i32)
                            n339 = global read "断电保存全局.vi" "MN"() -> (w381:string)
                            n340 = global read "断电保存全局.vi" "PW"() -> (w380:string)
                            n341 = Search and Replace String(input string=w373, search string="." ("搜索字符串")) -> (result string=w371:string)  [unwired: 6 in, 3 out]
                            n342 = call "数据编码.vi"("table输入"="实时数据" ("新元素/子数组"), "QN"=w371, "MN"=w381, "PW"=w380) -> ("错误常量"=w382:errorcluster, "通讯包字符串"=w384:string)  [unwired: 10 in]
                            n343 = global write "全局1.vi" "发送报文显示"(w384) -> ()
                            n344 = Greater Or Equal?(x=w378, y=w379) -> (x >= y?=w377:bool)
                            n345 = call "通信状态入队列.vi"("错误输入（无错误）"=w382, "枚举"=enum16{"打开连接", "发送数据", "读取数据", "数据处理", "关闭连接"}."发送数据") -> ()  [unwired: 9 in, 1 out]
                            n346 = Wait (ms)(milliseconds to wait=u32 1000 ("等待时间（毫秒）")) -> ()  [unwired: 1 out]
                          }
                        }
                      }
                    }
                    frame True {
                    }
                  }
                }
              }
            }
          }
        }
      }
      frame "操作日志" {
        # "间隔时间上传"
        # "直接1分钟查询 一次,有数据就按数据上传,没数据就不上传,在数据发送那边有做处理"
        n347 = flat-sequence {
          frame #0 {
            # "时间"
            n348 = global write "全局 小时数据发送次数.vi" "小时数据发送次数"(0 ("小时数据发送次数")) -> ()
            n349 = call "日志信息主动发送(子VI).vi"() -> ()  [unwired: 12 in]
            n350 = global write "全局1.vi" "枚举"(enum16{"返回请求应答", "上传数据", "返回执行结果"}."上传数据" ("枚举")) -> ()
          }
          frame #1 {
            n351 = call "获取操作日志 (子VI).vi"("table输入"="操作日志") -> ()  [unwired: 11 in]
          }
          frame #2 {
            n352 = global read "全局 数据发送重叠.vi" "掉线指示灯"() -> (w391:bool)
            n353 = Not(x=w391) -> (.not. x?=w390:bool)
            n354 = case shown="真" w390 {
              frame False {
              }
              frame True {
                n355 = global read "全局 时间2.vi" "仪器日志索引"() -> (w395:T13)
                n356 = Cluster To Array(cluster=w395) -> (array=w394:string[])
                n357 = for {
                  tunnel: w394 -> [w396] mode=indexing
                  tunnel: [w397] -> w392 mode=indexing
                  i -> [w399]
                  # "行数大于零"
                  n358 = case shown="5" w399 {
                    tunnel: [w403 w404 w405 w406 w407 w408] -> w398
                    frame 0, Default {
                      n359 = global read "全局 所有参数.vi" "氨氮"() -> (w403:string[][])
                    }
                    frame 1 {
                      n360 = global read "全局 所有参数.vi" "总磷"() -> (w404:string[][])
                    }
                    frame 2 {
                      n361 = global read "全局 所有参数.vi" "总氮"() -> (w405:string[][])
                    }
                    frame 3 {
                      n362 = global read "全局 所有参数.vi" "CODMn"() -> (w406:string[][])
                    }
                    frame 4 {
                      n363 = global read "全局 所有参数.vi" "CODCr"() -> (w407:string[][])
                    }
                    frame 5 {
                      n364 = global read "全局 所有参数.vi" "DO"() -> (w408:string[][])
                    }
                  }
                  n365 = Array Size(array=w398) -> (size(s)=w401:i32[])
                  n366 = Index Array(array=w401) -> (element=w400:i32)  [unwired: 1 in]
                  n367 = Greater Than 0?(x=w400) -> (x > 0?=w402:bool)
                  n368 = case shown="真" w402 {
                    tunnel: w400 -> [_ _]
                    tunnel: w398 -> [_ w414]
                    tunnel: [w409 w410] -> w397
                    tunnel: w396 -> [w409 _]
                    frame False {
                    }
                    frame True {
                      # "最新时间戳加1分钟"
                      n369 = Array Size(array=w414) -> (size(s)=w416:i32[])
                      n370 = Index Array(array=w416) -> (element=w415:i32)  [unwired: 1 in]
                      n371 = Decrement(x=w415) -> (x-1=w413:i32)
                      n372 = Index Array(array=w414, index (row)=w413, index (col)=0 ("禁用的索引 (列)")) -> (element=w411:string)
                      n373 = call "日期时间字符串转换秒数加一.vi"("data[0]"=w411) -> ("日期/时间字符串"=w410:string)  [unwired: 10 in]
                    }
                  }
                }
                n374 = Array To Cluster(array=w392) -> (cluster=w393:T14)
                n375 = global write "全局 时间2.vi" "仪器日志索引"(w393) -> ()
              }
            }
          }
          frame #3 {
            n376 = call "数据处理整合 (子VI).vi"("枚举"=enum16{"实时数据排序", "小时数据排序"}."实时数据排序") -> ("已排序的数组"=w419:string[])  [unwired: 10 in]
            n377 = Array Size(array=w419) -> (size(s)=w418:i32)
            n378 = global write "全局 数据数组大小.vi" "数据数组大小"(w418) -> ()
          }
          frame #4 {
            # "判定是否存表"
            n379 = global read "全局 数据发送重叠.vi" "掉线指示灯"() -> (w420:bool)
            n380 = case shown="假" w420 {
              frame False {
                n381 = global read "全局 数据数组大小.vi" "数据数组大小"() -> (w421:i32)
                n382 = Greater Than 0?(x=w421) -> (x > 0?=w422:bool)
                n383 = case shown="真" w422 {
                  frame False {
                  }
                  frame True {
                    n384 = while {
                      stop <- w424 stop-if-true
                      n385 = Get Date/Time In Seconds() -> (seconds since 1Jan1904=w436:timestamp)
                      n386 = Format Date/Time String(time format string (%c)="%Y%m%d%H%M%S%3u" ("时间格式字符串(%c)"), seconds (now)=w436) -> (date/time string=w435:string)  [unwired: 1 in]
                      n387 = Search and Replace String(input string=w435, search string="." ("搜索字符串")) -> (result string=w433:string)  [unwired: 6 in, 3 out]
                      n388 = global read "断电保存全局.vi" "MN"() -> (w430:string)
                      n389 = global read "断电保存全局.vi" "PW"() -> (w429:string)
                      n390 = call "数据编码.vi"("table输入"="操作日志" ("新元素/子数组"), "QN"=w433, "MN"=w430, "PW"=w429) -> ("错误常量"=w428:errorcluster, "通讯包字符串"=w432:string)  [unwired: 10 in]
                      n391 = global read "全局 小时数据发送次数.vi" "小时数据发送次数"() -> (w425:i32)
                      n392 = global read "全局 数据数组大小.vi" "数据数组大小"() -> (w426:i32)
                      n393 = call "通信状态入队列.vi"("错误输入（无错误）"=w428, "枚举"=enum16{"打开连接", "发送数据", "读取数据", "数据处理", "关闭连接"}."发送数据") -> ()  [unwired: 9 in, 1 out]
                      n394 = global write "全局1.vi" "发送报文显示"(w432) -> ()
                      n395 = Decrement(x=w426) -> (x-1=w427:i32)
                      n396 = Greater Or Equal?(x=w425, y=w427) -> (x >= y?=w424:bool)
                      n397 = Wait (ms)(milliseconds to wait=u32 1000 ("等待时间（毫秒）")) -> ()  [unwired: 1 out]
                    }
                  }
                }
              }
              frame True {
              }
            }
          }
        }
      }
      frame "仪器参数" {
        # "间隔时间上传"
        # "直接1分钟查询 一次,有数据就按数据上传,没数据就不上传,在数据发送那边有做处理"
        n398 = flat-sequence {
          frame #0 {
            n399 = global write "全局 小时数据发送次数.vi" "小时数据发送次数"(0 ("小时数据发送次数")) -> ()
            n400 = global write "全局1.vi" "枚举"(enum16{"返回请求应答", "上传数据", "返回执行结果"}."上传数据" ("枚举")) -> ()
          }
          frame #1 {
            n401 = call "获取操作日志 (子VI).vi"("table输入"="仪器参数") -> ()  [unwired: 11 in]
          }
          frame #2 {
            n402 = global read "全局 数据发送重叠.vi" "掉线指示灯"() -> (w444:bool)
            n403 = Not(x=w444) -> (.not. x?=w443:bool)
            n404 = case shown="真" w443 {
              frame False {
              }
              frame True {
                n405 = global read "全局 时间2.vi" "仪器参数索引"() -> (w448:T15)
                n406 = Cluster To Array(cluster=w448) -> (array=w447:string[])
                n407 = for {
                  tunnel: [w452] -> w445 mode=indexing
                  tunnel: w447 -> [w451] mode=indexing
                  i -> [w450]
                  # "行数大于零"
                  n408 = case shown="12" w450 {
                    tunnel: [w456 w457 w458 w459 w460 w461 w462 w463 w464 w465 w466 w467 w468] -> w449
                    frame 0, Default {
                      n409 = global read "全局 所有参数.vi" "氨氮"() -> (w456:string[][])
                    }
                    frame 1 {
                      n410 = global read "全局 所有参数.vi" "总磷"() -> (w457:string[][])
                    }
                    frame 2 {
                      n411 = global read "全局 所有参数.vi" "总氮"() -> (w458:string[][])
                    }
                    frame 3 {
                      n412 = global read "全局 所有参数.vi" "CODMn"() -> (w459:string[][])
                    }
                    frame 4 {
                      n413 = global read "全局 所有参数.vi" "CODCr"() -> (w460:string[][])
                    }
                    frame 5 {
                      n414 = global read "全局 所有参数.vi" "DO"() -> (w461:string[][])
                    }
                    frame 6 {
                      n415 = global read "全局 所有参数.vi" "PH"() -> (w462:string[][])
                    }
                    frame 7 {
                      n416 = global read "全局 所有参数.vi" "电导率"() -> (w463:string[][])
                    }
                    frame 8 {
                      n417 = global read "全局 所有参数.vi" "水温"() -> (w464:string[][])
                    }
                    frame 9 {
                      n418 = global read "全局 所有参数.vi" "浊度"() -> (w465:string[][])
                    }
                    frame 10 {
                      n419 = global read "全局 所有参数.vi" "叶绿素"() -> (w466:string[][])
                    }
                    frame 11 {
                      n420 = global read "全局 所有参数.vi" "藻密度"() -> (w467:string[][])
                    }
                    frame 12 {
                      n421 = global read "全局 所有参数.vi" "ORP"() -> (w468:string[][])
                    }
                  }
                  n422 = Array Size(array=w449) -> (size(s)=w454:i32[])
                  n423 = Index Array(array=w454) -> (element=w453:i32)  [unwired: 1 in]
                  n424 = Greater Than 0?(x=w453) -> (x > 0?=w455:bool)
                  n425 = case shown="真" w455 {
                    tunnel: w453 -> [_ _]
                    tunnel: w449 -> [_ w473]
                    tunnel: [w469 w470] -> w452
                    tunnel: w451 -> [w469 _]
                    frame False {
                    }
                    frame True {
                      # "最新时间戳加1分钟"
                      n426 = Array Size(array=w473) -> (size(s)=w475:i32[])
                      n427 = Index Array(array=w475) -> (element=w474:i32)  [unwired: 1 in]
                      n428 = Decrement(x=w474) -> (x-1=w472:i32)
                      n429 = Index Array(array=w473, index (row)=w472, index (col)=0 ("禁用的索引 (列)")) -> (element=w476:string)
                      n430 = call "日期时间字符串转换分钟数加一.vi"("data[0]"=w476) -> ("日期/时间字符串"=w470:string)  [unwired: 10 in]
                    }
                  }
                }
                n431 = Array To Cluster(array=w445) -> (cluster=w446:T16)
                n432 = global write "全局 时间2.vi" "仪器参数索引"(w446) -> ()
              }
            }
          }
          frame #3 {
            n433 = call "数据处理整合 (子VI).vi"("枚举"=enum16{"实时数据排序", "小时数据排序"}."实时数据排序") -> ("已排序的数组"=w479:string[])  [unwired: 10 in]
            n434 = Array Size(array=w479) -> (size(s)=w478:i32)
            n435 = global write "全局 数据数组大小.vi" "数据数组大小"(w478) -> ()
          }
          frame #4 {
            # "判定是否存表"
            n436 = global read "全局 数据发送重叠.vi" "掉线指示灯"() -> (w480:bool)
            n437 = case shown="假" w480 {
              frame False {
                n438 = global read "全局 数据数组大小.vi" "数据数组大小"() -> (w481:i32)
                n439 = Greater Than 0?(x=w481) -> (x > 0?=w482:bool)
                n440 = case shown="真" w482 {
                  frame False {
                  }
                  frame True {
                    n441 = while {
                      stop <- w483 stop-if-true
                      n442 = Get Date/Time In Seconds() -> (seconds since 1Jan1904=w496:timestamp)
                      n443 = Format Date/Time String(time format string (%c)="%Y%m%d%H%M%S%3u" ("时间格式字符串(%c)"), seconds (now)=w496) -> (date/time string=w495:string)  [unwired: 1 in]
                      n444 = Search and Replace String(input string=w495, search string="." ("搜索字符串")) -> (result string=w493:string)  [unwired: 6 in, 3 out]
                      n445 = global read "断电保存全局.vi" "MN"() -> (w490:string)
                      n446 = global read "断电保存全局.vi" "PW"() -> (w489:string)
                      n447 = global read "全局 数据数组大小.vi" "数据数组大小"() -> (w485:i32)
                      n448 = call "数据编码.vi"("table输入"="仪器参数" ("新元素/子数组"), "QN"=w493, "MN"=w490, "PW"=w489) -> ("错误常量"=w488:errorcluster, "通讯包字符串"=w492:string)  [unwired: 10 in]
                      n449 = global read "全局 小时数据发送次数.vi" "小时数据发送次数"() -> (w486:i32)
                      n450 = global write "全局1.vi" "发送报文显示"(w492) -> ()
                      n451 = call "通信状态入队列.vi"("错误输入（无错误）"=w488, "枚举"=enum16{"打开连接", "发送数据", "读取数据", "数据处理", "关闭连接"}."发送数据") -> ()  [unwired: 9 in, 1 out]
                      n452 = Decrement(x=w485) -> (x-1=w484:i32)
                      n453 = Greater Or Equal?(x=w486, y=w484) -> (x >= y?=w483:bool)
                      n454 = Wait (ms)(milliseconds to wait=u32 1000 ("等待时间（毫秒）")) -> ()  [unwired: 1 out]
                    }
                  }
                }
              }
              frame True {
              }
            }
          }
        }
      }
      frame "系统状态" {
        # "直接1分钟查询 一次,有变化就按上传,没变化就不上传"
        n455 = flat-sequence {
          frame #0 {
            # "时间"
            n456 = global write "全局 小时数据发送次数.vi" "小时数据发送次数"(0 ("小时数据发送次数")) -> ()
            n457 = global write "全局 数据数组大小.vi" "数据数组大小"(1 ("数据数组大小")) -> ()
            n458 = global write "全局1.vi" "枚举"(enum16{"返回请求应答", "上传数据", "返回执行结果"}."上传数据" ("枚举")) -> ()
          }
          frame #1 {
            # "判定是否存表"
            n459 = global read "全局 数据发送重叠.vi" "掉线指示灯"() -> (w503:bool)
            n460 = case shown="假" w503 {
              frame False {
                n461 = global read "全局1.vi" "系统状态"() -> (w504:bool)
                n462 = case shown="真" w504 {
                  frame False {
                  }
                  frame True {
                    n463 = global read "全局 小时数据发送次数.vi" "小时数据发送次数"() -> (w512:i32)
                    n464 = global write "全局1.vi" "系统状态"(FALSE ("系统状态")) -> ()
                    n465 = Get Date/Time In Seconds() -> (seconds since 1Jan1904=w516:timestamp)
                    n466 = Increment(x=w512) -> (x+1=w511:i32)
                    n467 = Format Date/Time String(time format string (%c)="%Y%m%d%H%M%S%3u" ("时间格式字符串(%c)"), seconds (now)=w516) -> (date/time string=w515:string)  [unwired: 1 in]
                    n468 = global write "全局 小时数据发送次数.vi" "小时数据发送次数"(w511) -> ()
                    n469 = Search and Replace String(input string=w515, search string="." ("搜索字符串")) -> (result string=w513:string)  [unwired: 6 in, 3 out]
                    n470 = global read "断电保存全局.vi" "MN"() -> (w508:string)
                    n471 = global read "断电保存全局.vi" "PW"() -> (w507:string)
                    n472 = call "数据编码.vi"("table输入"="系统状态" ("新元素/子数组"), "QN"=w513, "MN"=w508, "PW"=w507) -> ("错误常量"=w506:errorcluster, "通讯包字符串"=w510:string)  [unwired: 10 in]
                    n473 = call "通信状态入队列.vi"("错误输入（无错误）"=w506, "枚举"=enum16{"打开连接", "发送数据", "读取数据", "数据处理", "关闭连接"}."发送数据") -> ()  [unwired: 9 in, 1 out]
                    n474 = global write "全局1.vi" "发送报文显示"(w510) -> ()
                  }
                }
              }
              frame True {
              }
            }
          }
        }
      }
      frame "运行模式" {
        # "直接1分钟查询 一次,有变化就按上传,没变化就不上传"
        n475 = flat-sequence {
          frame #0 {
            # "时间"
            n476 = global write "全局 小时数据发送次数.vi" "小时数据发送次数"(0 ("小时数据发送次数")) -> ()
            n477 = global write "全局 数据数组大小.vi" "数据数组大小"(1 ("数据数组大小")) -> ()
            n478 = global write "全局1.vi" "枚举"(enum16{"返回请求应答", "上传数据", "返回执行结果"}."上传数据" ("枚举")) -> ()
          }
          frame #1 {
            # "判定是否存表"
            n479 = global read "全局 数据发送重叠.vi" "掉线指示灯"() -> (w523:bool)
            n480 = case shown="假" w523 {
              frame False {
                n481 = global read "全局1.vi" "运行模式"() -> (w524:bool)
                n482 = case shown="真" w524 {
                  frame False {
                  }
                  frame True {
                    n483 = global read "全局 小时数据发送次数.vi" "小时数据发送次数"() -> (w532:i32)
                    n484 = global write "全局1.vi" "运行模式"(FALSE ("系统状态")) -> ()
                    n485 = Get Date/Time In Seconds() -> (seconds since 1Jan1904=w536:timestamp)
                    n486 = Increment(x=w532) -> (x+1=w531:i32)
                    n487 = Format Date/Time String(time format string (%c)="%Y%m%d%H%M%S%3u" ("时间格式字符串(%c)"), seconds (now)=w536) -> (date/time string=w535:string)  [unwired: 1 in]
                    n488 = global write "全局 小时数据发送次数.vi" "小时数据发送次数"(w531) -> ()
                    n489 = Search and Replace String(input string=w535, search string="." ("搜索字符串")) -> (result string=w533:string)  [unwired: 6 in, 3 out]
                    n490 = global read "断电保存全局.vi" "MN"() -> (w528:string)
                    n491 = global read "断电保存全局.vi" "PW"() -> (w527:string)
                    n492 = call "数据编码.vi"("table输入"="运行模式" ("新元素/子数组"), "QN"=w533, "MN"=w528, "PW"=w527) -> ("错误常量"=w526:errorcluster, "通讯包字符串"=w530:string)  [unwired: 10 in]
                    n493 = call "通信状态入队列.vi"("错误输入（无错误）"=w526, "枚举"=enum16{"打开连接", "发送数据", "读取数据", "数据处理", "关闭连接"}."发送数据") -> ()  [unwired: 9 in, 1 out]
                    n494 = global write "全局1.vi" "发送报文显示"(w530) -> ()
                  }
                }
              }
              frame True {
              }
            }
          }
        }
      }
      frame "测量周期" {
        # "直接1分钟查询 一次,有变化就按上传,没变化就不上传"
        n495 = flat-sequence {
          frame #0 {
            # "时间"
            n496 = global write "全局 小时数据发送次数.vi" "小时数据发送次数"(0 ("小时数据发送次数")) -> ()
            n497 = global write "全局 数据数组大小.vi" "数据数组大小"(1 ("数据数组大小")) -> ()
            n498 = global write "全局1.vi" "枚举"(enum16{"返回请求应答", "上传数据", "返回执行结果"}."上传数据" ("枚举")) -> ()
          }
          frame #1 {
            # "判定是否存表"
            n499 = global read "全局 数据发送重叠.vi" "掉线指示灯"() -> (w543:bool)
            n500 = case shown="假" w543 {
              frame False {
                n501 = global read "全局1.vi" "测量周期"() -> (w544:bool)
                n502 = case shown="真" w544 {
                  frame False {
                  }
                  frame True {
                    n503 = global read "全局 小时数据发送次数.vi" "小时数据发送次数"() -> (w552:i32)
                    n504 = global write "全局1.vi" "测量周期"(FALSE ("系统状态")) -> ()
                    n505 = Get Date/Time In Seconds() -> (seconds since 1Jan1904=w556:timestamp)
                    n506 = Increment(x=w552) -> (x+1=w551:i32)
                    n507 = Format Date/Time String(time format string (%c)="%Y%m%d%H%M%S%3u" ("时间格式字符串(%c)"), seconds (now)=w556) -> (date/time string=w555:string)  [unwired: 1 in]
                    n508 = global write "全局 小时数据发送次数.vi" "小时数据发送次数"(w551) -> ()
                    n509 = Search and Replace String(input string=w555, search string="." ("搜索字符串")) -> (result string=w553:string)  [unwired: 6 in, 3 out]
                    n510 = global read "断电保存全局.vi" "MN"() -> (w548:string)
                    n511 = global read "断电保存全局.vi" "PW"() -> (w547:string)
                    n512 = call "数据编码.vi"("table输入"="测量周期" ("新元素/子数组"), "QN"=w553, "MN"=w548, "PW"=w547) -> ("错误常量"=w546:errorcluster, "通讯包字符串"=w550:string)  [unwired: 10 in]
                    n513 = global write "全局1.vi" "发送报文显示"(w550) -> ()
                    n514 = call "通信状态入队列.vi"("错误输入（无错误）"=w546, "枚举"=enum16{"打开连接", "发送数据", "读取数据", "数据处理", "关闭连接"}."发送数据") -> ()  [unwired: 9 in, 1 out]
                  }
                }
              }
              frame True {
              }
            }
          }
        }
      }
      frame "超标留样" {
        # "直接1分钟查询 一次,有变化就按上传,没变化就不上传"
        n515 = flat-sequence {
          frame #0 {
            # "时间"
            n516 = global write "全局 小时数据发送次数.vi" "小时数据发送次数"(0 ("小时数据发送次数")) -> ()
            n517 = global write "全局 数据数组大小.vi" "数据数组大小"(1 ("数据数组大小")) -> ()
            n518 = global write "全局1.vi" "枚举"(enum16{"返回请求应答", "上传数据", "返回执行结果"}."上传数据" ("枚举")) -> ()
          }
          frame #1 {
            # "判定是否存表"
            n519 = global read "全局 数据发送重叠.vi" "掉线指示灯"() -> (w563:bool)
            n520 = case shown="假" w563 {
              frame False {
                n521 = global read "全局1.vi" "超标留样"() -> (w564:bool)
                n522 = case shown="真" w564 {
                  frame False {
                  }
                  frame True {
                    n523 = global read "全局 小时数据发送次数.vi" "小时数据发送次数"() -> (w572:i32)
                    n524 = global write "全局1.vi" "超标留样"(FALSE ("系统状态")) -> ()
                    n525 = Get Date/Time In Seconds() -> (seconds since 1Jan1904=w576:timestamp)
                    n526 = Increment(x=w572) -> (x+1=w571:i32)
                    n527 = Format Date/Time String(time format string (%c)="%Y%m%d%H%M%S%3u" ("时间格式字符串(%c)"), seconds (now)=w576) -> (date/time string=w575:string)  [unwired: 1 in]
                    n528 = global write "全局 小时数据发送次数.vi" "小时数据发送次数"(w571) -> ()
                    n529 = Search and Replace String(input string=w575, search string="." ("搜索字符串")) -> (result string=w573:string)  [unwired: 6 in, 3 out]
                    n530 = global read "断电保存全局.vi" "MN"() -> (w567:string)
                    n531 = global read "断电保存全局.vi" "PW"() -> (w566:string)
                    n532 = call "数据编码.vi"("table输入"="超标留样" ("新元素/子数组"), "QN"=w573, "MN"=w567, "PW"=w566) -> ("错误常量"=w568:errorcluster, "通讯包字符串"=w570:string)  [unwired: 10 in]
                    n533 = global write "全局1.vi" "发送报文显示"(w570) -> ()
                    n534 = call "通信状态入队列.vi"("错误输入（无错误）"=w568, "枚举"=enum16{"打开连接", "发送数据", "读取数据", "数据处理", "关闭连接"}."发送数据") -> ()  [unwired: 9 in, 1 out]
                  }
                }
              }
              frame True {
              }
            }
          }
        }
      }
      frame "报警信息" {
        # "间隔时间上传"
        # "直接1分钟查询 一次,有数据就按数据上传,没数据为空的不传,在数据发送那边有做处理"
        n535 = flat-sequence {
          frame #0 {
            # "分钟时间间隔"
            n536 = call "日志信息主动发送(子VI).vi"() -> ()  [unwired: 12 in]
            n537 = global write "全局 小时数据发送次数.vi" "小时数据发送次数"(0 ("小时数据发送次数")) -> ()
            n538 = global write "全局1.vi" "枚举"(enum16{"返回请求应答", "上传数据", "返回执行结果"}."上传数据" ("枚举")) -> ()
          }
          frame #1 {
            n539 = call "获取报警信息 (子VI).vi"() -> ()  [unwired: 12 in]
          }
          frame #2 {
            n540 = global read "全局 数据发送重叠.vi" "掉线指示灯"() -> (w583:bool)
            n541 = Not(x=w583) -> (.not. x?=w582:bool)
            n542 = case shown="真" w582 {
              frame False {
              }
              frame True {
                n543 = global read "全局 时间2.vi" "报警信息索引"() -> (w587:T17)
                n544 = Cluster To Array(cluster=w587) -> (array=w586:string[])
                n545 = for {
                  tunnel: [w589] -> w584 mode=indexing
                  tunnel: w586 -> [w588] mode=indexing
                  i -> [w591]
                  # "行数大于零"
                  n546 = case shown="1" w591 {
                    tunnel: [w595 w596 w597 w598 w599 w600 w601 w602 w603 w604 w605 w606] -> w590
                    frame 0, Default {
                      n547 = global read "全局 所有参数.vi" "氨氮"() -> (w595:string[][])
                    }
                    frame 1 {
                      n548 = global read "全局 所有参数.vi" "总磷"() -> (w596:string[][])
                    }
                    frame 2 {
                      n549 = global read "全局 所有参数.vi" "总氮"() -> (w597:string[][])
                    }
                    frame 3 {
                      n550 = global read "全局 所有参数.vi" "CODMn"() -> (w598:string[][])
                    }
                    frame 4 {
                      n551 = global read "全局 所有参数.vi" "CODCr"() -> (w599:string[][])
                    }
                    frame 5 {
                      n552 = global read "全局 所有参数.vi" "DO"() -> (w600:string[][])
                    }
                    frame 6 {
                      n553 = global read "全局 所有参数.vi" "PH"() -> (w601:string[][])
                    }
                    frame 7 {
                      n554 = global read "全局 所有参数.vi" "电导率"() -> (w602:string[][])
                    }
                    frame 8 {
                      n555 = global read "全局 所有参数.vi" "水温"() -> (w603:string[][])
                    }
                    frame 9 {
                      n556 = global read "全局 所有参数.vi" "浊度"() -> (w604:string[][])
                    }
                    frame 10 {
                      n557 = global read "全局 所有参数.vi" "叶绿素"() -> (w605:string[][])
                    }
                    frame 11 {
                      n558 = global read "全局 所有参数.vi" "藻密度"() -> (w606:string[][])
                    }
                  }
                  n559 = Array Size(array=w590) -> (size(s)=w593:i32[])
                  n560 = Index Array(array=w593) -> (element=w592:i32)  [unwired: 1 in]
                  n561 = Greater Than 0?(x=w592) -> (x > 0?=w594:bool)
                  n562 = case shown="真" w594 {
                    tunnel: w592 -> [_ _]
                    tunnel: w590 -> [_ w611]
                    tunnel: [w607 w608] -> w589
                    tunnel: w588 -> [w607 _]
                    frame False {
                    }
                    frame True {
                      # "最新时间戳加1分钟"
                      n563 = Array Size(array=w611) -> (size(s)=w613:i32[])
                      n564 = Index Array(array=w613) -> (element=w612:i32)  [unwired: 1 in]
                      n565 = Decrement(x=w612) -> (x-1=w610:i32)
                      n566 = Index Array(array=w611, index (row)=w610, index (col)=0 ("禁用的索引 (列)")) -> (element=w614:string)
                      n567 = call "日期时间字符串转换分钟数加一.vi"("data[0]"=w614) -> ("日期/时间字符串"=w608:string)  [unwired: 10 in]
                    }
                  }
                }
                n568 = Array To Cluster(array=w584) -> (cluster=w585:T18)
                n569 = global write "全局 时间2.vi" "报警信息索引"(w585) -> ()
              }
            }
          }
          frame #3 {
            n570 = call "数据处理整合 (子VI).vi"("枚举"=enum16{"实时数据排序", "小时数据排序"}."实时数据排序") -> ("已排序的数组"=w617:string[])  [unwired: 10 in]
            n571 = Array Size(array=w617) -> (size(s)=w616:i32)
            n572 = global write "全局 数据数组大小.vi" "数据数组大小"(w616) -> ()
          }
          frame #4 {
            # "判定是否存表"
            n573 = global read "全局 数据发送重叠.vi" "掉线指示灯"() -> (w618:bool)
            n574 = case shown="假" w618 {
              frame False {
                # "判定数据不为空才发"
                n575 = global read "全局 数据数组大小.vi" "数据数组大小"() -> (w619:i32)
                n576 = Greater Than 0?(x=w619) -> (x > 0?=w620:bool)
                n577 = case shown="真" w620 {
                  frame False {
                    n578 = global write "全局1.vi" "核查数据上传"(FALSE ("数据上传")) -> ()
                  }
                  frame True {
                    n579 = while {
                      stop <- w623 stop-if-true
                      n580 = Wait (ms)(milliseconds to wait=u32 1000 ("等待时间（毫秒）")) -> ()  [unwired: 1 out]
                      n581 = Get Date/Time In Seconds() -> (seconds since 1Jan1904=w635:timestamp)
                      n582 = Format Date/Time String(time format string (%c)="%Y%m%d%H%M%S%3u" ("时间格式字符串(%c)"), seconds (now)=w635) -> (date/time string=w634:string)  [unwired: 1 in]
                      n583 = global read "全局 数据数组大小.vi" "数据数组大小"() -> (w625:i32)
                      n584 = Search and Replace String(input string=w634, search string="." ("搜索字符串")) -> (result string=w632:string)  [unwired: 6 in, 3 out]
                      n585 = global read "断电保存全局.vi" "MN"() -> (w629:string)
                      n586 = global read "断电保存全局.vi" "PW"() -> (w628:string)
                      n587 = global read "全局 小时数据发送次数.vi" "小时数据发送次数"() -> (w626:i32)
                      n588 = call "数据编码.vi"("table输入"="报警信息" ("新元素/子数组"), "QN"=w632, "MN"=w629, "PW"=w628) -> ("错误常量"=w627:errorcluster, "通讯包字符串"=w631:string)  [unwired: 10 in]
                      n589 = Decrement(x=w625) -> (x-1=w624:i32)
                      n590 = global write "全局1.vi" "发送报文显示"(w631) -> ()
                      n591 = Greater Or Equal?(x=w626, y=w624) -> (x >= y?=w623:bool)
                      n592 = call "通信状态入队列.vi"("错误输入（无错误）"=w627, "枚举"=enum16{"打开连接", "发送数据", "读取数据", "数据处理", "关闭连接"}."发送数据") -> ()  [unwired: 9 in, 1 out]
                    }
                  }
                }
              }
              frame True {
              }
            }
          }
        }
      }
      frame "环境参数" {
        n593 = call "核查数据断电保存 (子VI).vi"() -> ()  [unwired: 12 in]
      }
    }
    n594 = Not(x=w4) -> (.not. x?=w5:bool)
    n595 = global write "全局1.vi" "核查数据上传"(w5) -> ()
  }
  "错误输出" <- w1
